vi "更新文件.vi"(11 "服务器信息":T1={"host"="27.154.58.30", "user"="fb", "password"="std23506", "远端地址"="/725测试平台"}) -> ()   [LabVIEW 2016, in "update.lvlib"]
uses:
  update.lvlib
  <vilib>/FTP/ftp2.llb/FTP File Info.ctl
  <vilib>/FTP/NI_FTP.lvlib
panel:
  out "FTP链接结束":bool
  out "滑动杆":dbl(slide) scale=0.0..100.0
  out "大小":i64
  out "path info":T2={"type"=enum."link", "permissions"="", "owner"="", "group"="", "size"=0, "date"="", "name"="", "link name"=""} caption="路径信息"
  out "command":string caption="命令"
  out "last status string":string caption="最近状态字符串"
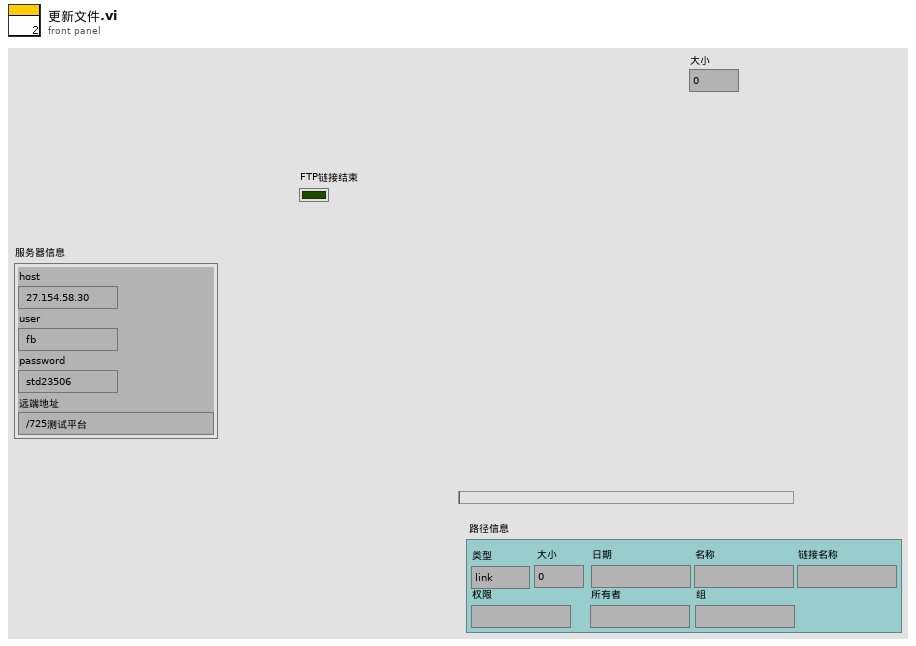
[diagram p1: front panel]
types:
  T1 = cluster{"host":string, "user":string, "password":string, "远端地址":string}
  T2 = typedef "NI_FTP.lvlib/FTP File Info.ctl" = cluster{"type":enum16{"unknown", "file", "dir", "link"}, "permissions":string, "owner":string, "group":string, "size":i32, "date":string, "name":string, "link name":string}
  T3 = cluster{"command":string, "last status string":string, dbl}
  T4 = cluster{"command":string, "last status string":string, "process":dbl}
  T5 = cluster{"remote path":string, "local path":path, "binary":bool}
  T6 = cluster{"remote path":string, "local path":path, "binary":bool}[]
  T7 = typedef "NI_FTP.lvlib/FTP Session.ctl" = refnum<k5>
  T8 = enum32{"invalid app kind", "Development System", "Run Time System", "Student Edition", "Embedded LabVIEW", "Evaluation", "Custom"}
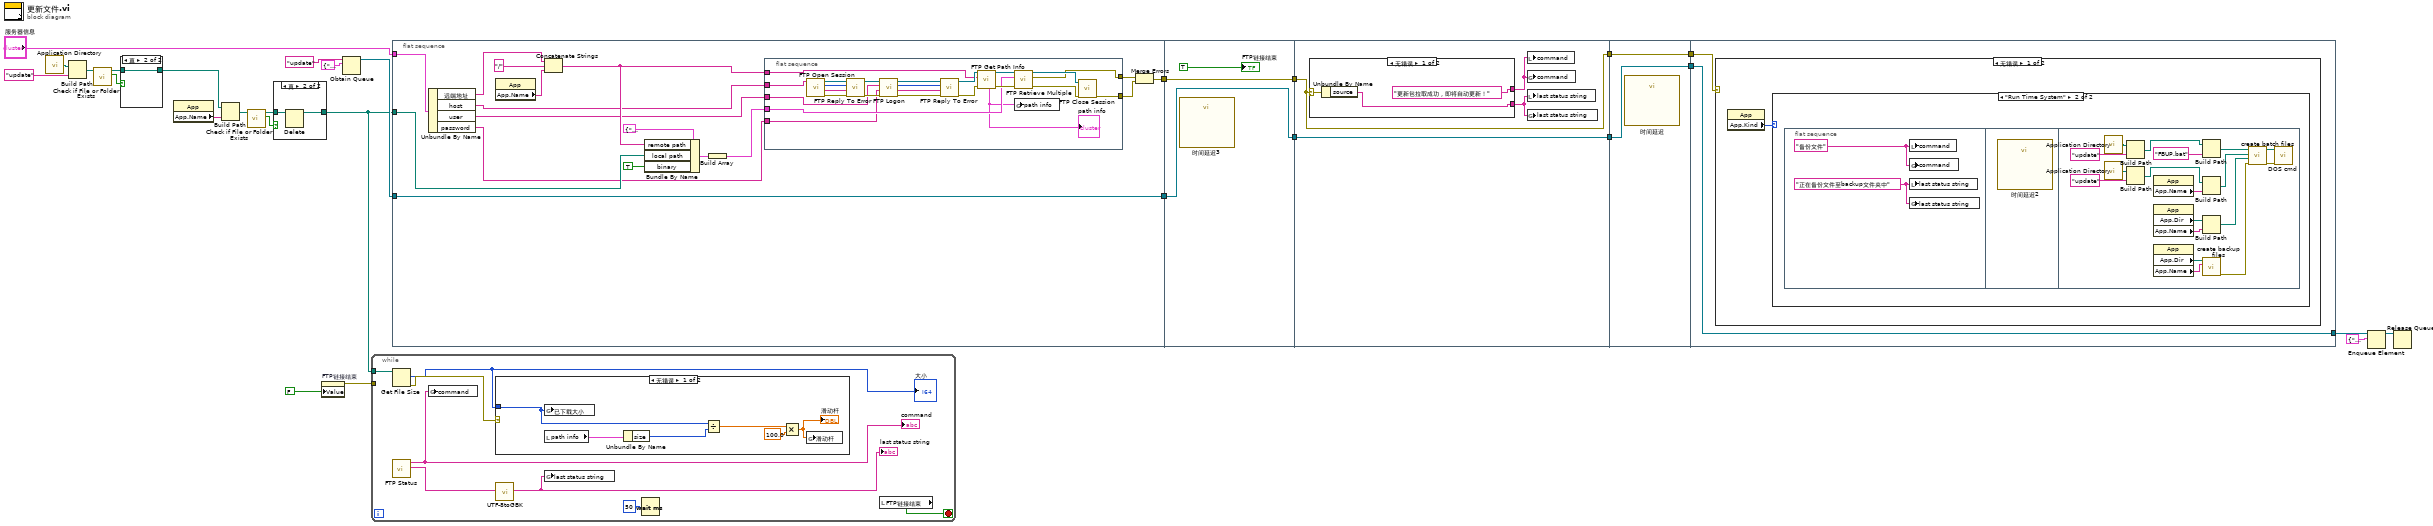
[diagram p0: block diagram]
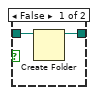
[diagram p4: hidden frame]
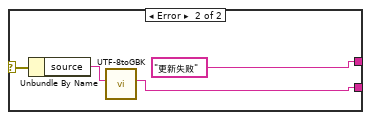
[diagram p5: hidden frame]
diagram:
  n1 = call <vilib>:"Application Directory.vi"() -> ("Application Directory"=w20:path)
  n2 = Build Path(base path=w20, name or relative path="update" ("名称或相对路径")) -> (appended path=w21:path)
  n3 = call <vilib>:"Check if File or Folder Exists.vi"("path"=w21) -> ("file or folder exists?"=w22:bool, "dup path"=w23:path)  [unwired: 8 in, 1 out]
  n4 = case shown="真" w22 {
    tunnel: w23 -> [w30 w31]
    tunnel: [w29 w31] -> w18
    frame False {
      n5 = Create Folder(path (use dialog)=w30) -> (created path=w29:path)  [unwired: 2 in, 2 out]
    }
    frame True {
    }
  }
  n6 = property class="App"() -> ("App.Name"=w2:string)  [unwired: 2 in, 2 out]
  n7 = Build Path(base path=w18, name or relative path=w2) -> (appended path=w17:path)
  n8 = call <vilib>:"Check if File or Folder Exists.vi"("path"=w17) -> ("file or folder exists?"=w16:bool, "dup path"=w15:path)  [unwired: 8 in, 1 out]
  n9 = case shown="真" w16 {
    tunnel: w15 -> [w32 w34]
    tunnel: [w32 w33] -> w13
    frame False {
    }
    frame True {
      n10 = Delete(path (use dialog)=w34) -> (deleted path=w33:path)  [unwired: 4 in, 2 out]
    }
  }
  n11 = property on="FTP链接结束" class="Bool (严格)"("Value"=FALSE ("FTP链接结束")) -> (error out=w12:errorcluster)  [unwired: 2 in, 1 out]
  n12 = Obtain Queue(name (unnamed)="update" ("名称（未命名）"), element data type=T4 {"command"="", "last status string"="", "process"=0.0}) -> (queue out=w14:refnum<queue>)  [unwired: 3 in, 2 out]
  n13 = while {
    tunnel: w13 -> [w39]
    tunnel: w12 -> [_]
    stop <- w35 stop-if-true
    n14 = Get File Size(file=w39) -> (size (in bytes)=w37:i64, 0:w38:errorcluster)  [unwired: 1 in, 1 out]
    "大小" <- w37
    n15 = call "FTP Status"() -> ("last status string"=w42:string, "command"=w41:string)  [unwired: 10 in]
    "command" <- w41
    n16 = global write "更新全局变量.vi" "command"(w41) -> ()
    n17 = case shown="无错误" w38 {
      tunnel: w37 -> [w44 _]
      frame No Error {
        n18 = global write "更新全局变量.vi" "已下载大小"(w44) -> ()
        n19 = local read "path info"() -> (w48:T2)
        n20 = Unbundle By Name(w48) -> ("size"=w47:i32)
        n21 = Divide(x=w44, y=w47) -> (x/y=w46:dbl)
        n22 = Multiply(x=w46, y=100.0) -> (x*y=w43:dbl)
        "滑动杆" <- w43
        n23 = global write "更新全局变量.vi" "滑动杆"(w43) -> ()
      }
      frame Error {
      }
    }
    n24 = call "UTF-8toGBK.vi"("UTF-8"=w42) -> ("GBK"=w40:string)  [unwired: 9 in, 1 out]
    "last status string" <- w40
    n25 = global write "更新全局变量.vi" "last status string"(w40) -> ()
    n26 = Wait (ms)(milliseconds to wait=u32 50 ("等待时间（毫秒）")) -> ()  [unwired: 1 out]
    n27 = local read "FTP链接结束"() -> (w35:bool)
  }
  n28 = flat-sequence {
    tunnel: [w65] -> w10
    tunnel: w14 -> [w63]
    tunnel: [w63] -> w8
    tunnel: w13 -> [w64]
    tunnel: "服务器信息" -> [w55]
    tunnel: w10 -> [w92]
    tunnel: [w92] -> w9
    tunnel: w8 -> [w91]
    tunnel: [w91] -> w7
    tunnel: w9 -> [w96]
    tunnel: [w96] -> w6
    tunnel: w7 -> [w93]
    tunnel: [w93] -> w4
    tunnel: w6 -> [w105]
    tunnel: [w105] -> w5
    tunnel: w4 -> [w104]
    tunnel: [w104] -> w3
    tunnel: w5 -> [w106]
    tunnel: w3 -> [w107]
    tunnel: [w107] -> w26
    frame #0 {
      n29 = Unbundle By Name(w55) -> ("远端地址"=w54:string, "host"=w53:string, "user"=w51:string, "password"=w52:string)
      n30 = property class="App"() -> ("App.Name"=w49:string)  [unwired: 2 in, 2 out]
      n31 = Concatenate Strings(w54, "/" ("remote path"), w49) -> (w56:string)
      n32 = Bundle By Name(cluster=T5 {"remote path"="", "local path"=path "", "binary"=FALSE} ("transfer spec"), "remote path"=w56, "local path"=w64, "binary"=TRUE) -> (w61:T5)
      n33 = Build Array(w61) -> (w59:T6)
      n34 = flat-sequence {
        tunnel: w59 -> [w73]
        tunnel: w56 -> [w72]
        tunnel: [w71] -> w58
        tunnel: [w70] -> w57
        tunnel: w53 -> [w68]
        tunnel: w52 -> [w67]
        tunnel: w51 -> [w66]
        frame #0 {
          n35 = call <vilib>:"FTP Open Session.vi"("address"=w68) -> ("error out"=w75:errorcluster, "reply string"=w77:string, "reply code"=w76:i32, "ftp session"=w74:T7)  [unwired: 3 in, 4 out]
          n36 = call <vilib>:"FTP Reply To Error.vi"("error in (no error)"=w75, "reply string in"=w77, "reply code in"=w76, "ftp session"=w74) -> ("error out"=w78:errorcluster, "ftp session out"=w79:T7)  [unwired: 2 out]
          n37 = call <vilib>:"FTP Logon.vi"("error in (no error)"=w78, "password"=w67, "user"=w66, "ftp session"=w79) -> ("error out"=w80:errorcluster, "reply string"=w82:string, "reply code"=w83:i32, "ftp session out"=w81:T7)  [unwired: 4 out]
          n38 = call <vilib>:"FTP Reply To Error.vi"("error in (no error)"=w80, "reply string in"=w82, "reply code in"=w83, "ftp session"=w81) -> ("error out"=w88:errorcluster, "ftp session out"=w86:T7)  [unwired: 2 out]
          n39 = call <vilib>:"FTP Get Path Info.vi"("error in (no error)"=w88, "remote path"=w72, "ftp session"=w86) -> ("error out"=w89:errorcluster, "ftp session out"=w87:T7, "path info"=w69:T2)  [unwired: 4 in, 2 out]
          "path info" <- w69
          n40 = call <vilib>:"FTP Retrieve Multiple.vi"("error in (no error)"=w89, "file specifications"=w73, "ftp session"=w87) -> ("error out"=w85:errorcluster, "file errors"=w71:errorcluster[], "ftp session out"=w84:T7)  [unwired: 2 in, 4 out]
          n41 = global write "更新全局变量.vi" "path info"(w69) -> ()
          n42 = call <vilib>:"FTP Close Session.vi"("error in (no error)"=w85, "ftp session"=w84) -> ("error out"=w70:errorcluster)  [unwired: 9 out]
        }
      }
      n43 = Merge Errors(w58, w57) -> (w65:errorcluster)
    }
    frame #1 {
      n44 = call "时间延迟3"() -> ()  [unwired: 11 in, 1 out]
      "FTP链接结束" <- TRUE ("FTP链接结束")
    }
    frame #2 {
      n45 = case shown="无错误" w96 {
        selector: w96 -> [w98 w103]
        tunnel: ["更新包拉取成功，即将自动更新！" ("command") "更新失败" ("command")] -> w95
        tunnel: [w97 w100] -> w94
        frame No Error {
          n46 = Unbundle By Name(w98) -> ("source"=w97:string)
        }
        frame Error {
          n47 = Unbundle By Name(w103) -> ("source"=w101:string)
          n48 = call "UTF-8toGBK.vi"("UTF-8"=w101) -> ("GBK"=w100:string)  [unwired: 9 in, 1 out]
        }
      }
      n49 = local write "command"(w95) -> ()
      n50 = global write "更新全局变量.vi" "command"(w95) -> ()
      n51 = local write "last status string"(w94) -> ()
      n52 = global write "更新全局变量.vi" "last status string"(w94) -> ()
    }
    frame #3 {
      n53 = call "时间延迟"() -> ()  [unwired: 11 in, 1 out]
    }
    frame #4 {
      n54 = case shown="无错误" w106 {
        frame No Error {
          n55 = property class="App"() -> ("App.Kind"=w108:T8)  [unwired: 2 in, 2 out]
          n56 = case shown="\"Run Time System\"" w108 {
            frame "invalid app kind", Default {
            }
            frame "Run Time System" {
              n57 = flat-sequence {
                frame #0 {
                  w109 = "正在备份文件至backup文件夹中" ("last status string")
                  w110 = "备份文件" ("command")
                  n58 = local write "command"(w110) -> ()
                  n59 = global write "更新全局变量.vi" "command"(w110) -> ()
                  n60 = local write "last status string"(w109) -> ()
                  n61 = global write "更新全局变量.vi" "last status string"(w109) -> ()
                }
                frame #1 {
                  n62 = call "时间延迟2"() -> ()  [unwired: 11 in, 1 out]
                }
                frame #2 {
                  n63 = call <vilib>:"Application Directory.vi"() -> ("Application Directory"=w114:path)
                  n64 = call <vilib>:"Application Directory.vi"() -> ("Application Directory"=w124:path)
                  n65 = Build Path(base path=w114, name or relative path="update" ("名称或相对路径")) -> (appended path=w115:path)
                  n66 = Build Path(base path=w124, name or relative path="update" ("名称或相对路径")) -> (appended path=w122:path)
                  n67 = property class="App"() -> ("App.Name"=w121:string)  [unwired: 2 in, 2 out]
                  n68 = property class="App"() -> ("App.Dir"=w120:path, "App.Name"=w119:string)  [unwired: 2 in, 2 out]
                  n69 = property class="App"() -> ("App.Dir"=w118:path, "App.Name"=w117:string)  [unwired: 2 in, 2 out]
                  n70 = Build Path(base path=w115, name or relative path="FBUP.bat" ("batch file name")) -> (appended path=w111:path)
                  n71 = Build Path(base path=w122, name or relative path=w121) -> (appended path=w113:path)
                  n72 = Build Path(base path=w120, name or relative path=w119) -> (appended path=w112:path)
                  n73 = call "create backup files.vi"("execute file name"=w117, "路径"=w118) -> ("error out"=w126:errorcluster)  [unwired: 9 in]
                  n74 = call "create batch files.vi"("错误输入（无错误）"=w126, "Targe Path"=w112, "Source Path"=w113, "Batch file"=w111) -> ("错误输出"=w127:errorcluster)  [unwired: 7 in]
                  n75 = call "DOS cmd.vi"("错误输入（无错误）"=w127, "批处理文件路径"=w111) -> ()  [unwired: 9 in, 1 out]
                }
              }
            }
          }
        }
        frame Error {
        }
      }
    }
  }
  n76 = Enqueue Element(queue=w26, element=T3 {"command"="stop", "last status string"="", 0.0} ("元素")) -> (queue out=w25:refnum<queue>)  [unwired: 2 in, 2 out]
  n77 = Release Queue(queue=w25) -> ()  [unwired: 2 in, 3 out]
